vi "RW Keywords Log File.vi"(8 "error in (no error)":errorcluster) -> (0 "error in (no error) 2":errorcluster)   [LabVIEW 2018]
uses:
  Log File/Log File.lvclass
  <vilib>/addons/_JKI Toolkits/Caraya/classes/Test/Test.lvclass
  <vilib>/addons/_JKI Toolkits/Caraya/classes/Assert/Assert.lvclass
  <vilib>/addons/_JKI Toolkits/Caraya/classes/Assert/Assert Equal Value_Variant.vi
  Keywords Log File/Keywords Log File.lvclass
  C:/Users/Denis/Desktop/S4ACS/S4ACS/Log File/Log File.lvclass
panel:
  in  "file refnum":refnum<file>
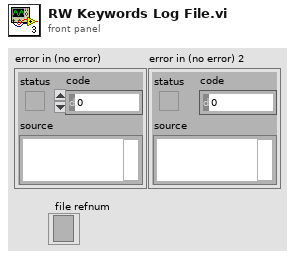
[diagram p1: front panel]
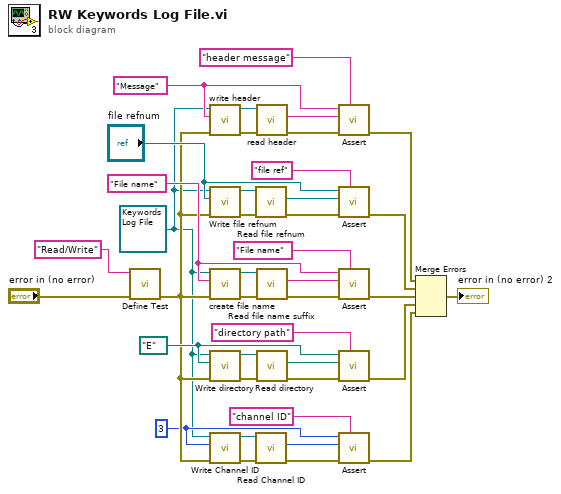
[diagram p0: block diagram]
diagram:
  w1 = refnum<class "Keywords Log File.lvclass"> refnum ("Keywords Log File.lvclass")
  w6 = u8 3 ("Channel ID")
  w15 = path "E:/" ("directory")
  w19 = "File name" ("file name")
  w34 = "Message" ("Label (VI Title)")
  n1 = call <vilib>:"Define Test.vi"("error in (no error)"="error in (no error)", "Label (VI Title)"="Read/Write") -> ("error out"=w8:errorcluster)  [unwired: 8 in, 1 out]
  n2 = call "write header.vi"("error in (no error)"=w8, "header"=w34, "Log File in"=w1) -> ("error out"=w37:errorcluster, "Log File out"=w38:refnum<class "Keywords Log File.lvclass">)  [unwired: 7 in]
  n3 = call "Write file refnum.vi"("error in (no error)"=w8, "file refnum"="file refnum", "Log File in"=w1) -> ("error out"=w30:errorcluster, "Log File out"=w28:refnum<class "Keywords Log File.lvclass">)  [unwired: 7 in]
  n4 = call "create file name.vi"("error in (no error)"=w8, 10:w19, "Log File in"=w1) -> ("error out"=w20:errorcluster, "Log File out"=w21:refnum<class "Keywords Log File.lvclass">)  [unwired: 7 in]
  n5 = call "Write directory.vi"("error in (no error)"=w8, "log dir"=w15, "Log File in"=w1) -> ("error out"=w18:errorcluster, "Log File out"=w17:refnum<class "Keywords Log File.lvclass">)  [unwired: 7 in]
  n6 = call "Write Channel ID.vi"("error in (no error)"=w8, "Channel ID"=w6, "Log File in"=w1) -> ("error out"=w11:errorcluster, "Log File out"=w10:refnum<class "Keywords Log File.lvclass">)  [unwired: 7 in]
  n7 = call "Read file refnum.vi"("error in (no error)"=w30, "Log File in"=w28) -> ("error out"=w29:errorcluster, "file refnum"=w27:refnum<file>)  [unwired: 7 in, 1 out]
  n8 = call "Read Channel ID.vi"("error in (no error)"=w11, "Log File in"=w10) -> ("error out"=w9:errorcluster, "Channel ID"=w7:u8)  [unwired: 7 in, 1 out]
  n9 = call "read header.vi"("error in (no error)"=w37, "Log File in"=w38) -> ("error out"=w36:errorcluster, "header"=w35:string)  [unwired: 7 in, 1 out]
  n10 = call "Read file name suffix.vi"("error in (no error)"=w20, "Log File in"=w21) -> ("error out"=w23:errorcluster, "file name"=w22:string)  [unwired: 7 in, 1 out]
  n11 = call "Read directory.vi"("error in (no error)"=w18, "Log File in"=w17) -> ("error out"=w14:errorcluster, "directory"=w16:path)  [unwired: 7 in, 1 out]
  n12 = call-poly <vilib>:"Assert.vi"("Label"="header message", "error in (no error)"=w36, "Actual"=w35, "Expected"=w34) -> ("error out"=w33:errorcluster)  [unwired: 6 in, 1 out]
  n13 = call-poly <vilib>:"Assert.vi"("Label"="file ref", "error in (no error)"=w29, "Actual"=w27, "Expected"="file refnum") -> ("error out"=w25:errorcluster)  [unwired: 6 in, 1 out]
  n14 = call-poly <vilib>:"Assert.vi"("Label"="File name" ("file name"), "error in (no error)"=w23, "Actual"=w22, "Expected"=w19) -> ("error out"=w4:errorcluster)  [unwired: 6 in, 1 out]
  n15 = call-poly <vilib>:"Assert.vi"("Label"="directory path" ("file name"), "error in (no error)"=w14, "Actual"=w16, "Expected"=w15) -> ("error out"=w3:errorcluster)  [unwired: 6 in, 1 out]
  n16 = call-poly <vilib>:"Assert.vi"("Label"="channel ID" ("file name"), "error in (no error)"=w9, "Actual"=w7, "Expected"=w6) -> ("error out"=w2:errorcluster)  [unwired: 6 in, 1 out]
  n17 = Merge Errors(w33, w25, w4, w3, w2) -> (→"error in (no error) 2":errorcluster)
